vi "ep_Detect Signaling Voltage.vi"(7 "signaling frequency":dbl=216.66, 8 "error in (no error)":errorcluster, 10 "current spectrum (5Hz step)":T2, 11 "voltage spectrum (5Hz step)":T2) -> (0 "error out":errorcluster, 1 "detected signaling frequency [Hz]":dbl, 2 "signaling current RMS [A]":dbl, 3 "signaling voltage RMS [V]":dbl)   [LabVIEW 2014, in "NI_EP_Power Quality.lvlib"]
uses:
  <vilib>/addons/Electrical Power/PQ/NI_EP_Power Quality.lvlib
  <vilib>/addons/Electrical Power/PQ/Common/Controls/ep_AI Data Channel.ctl
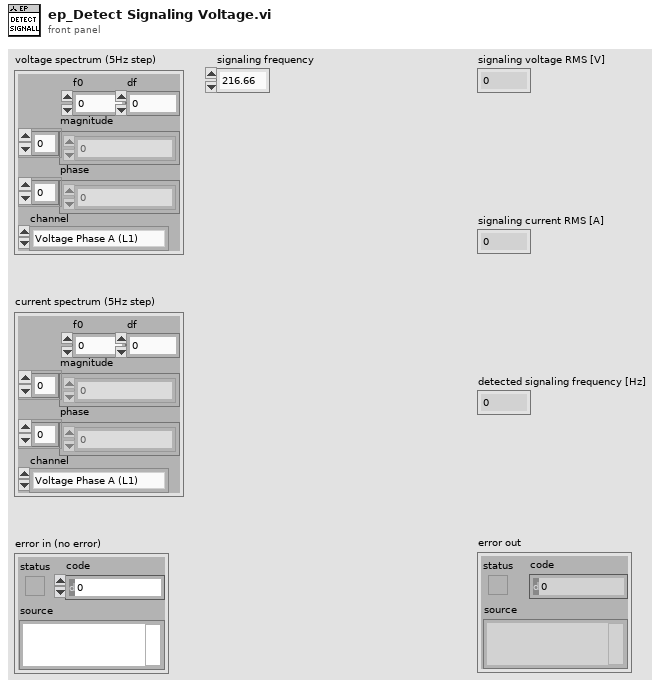
[diagram p1: front panel]
types:
  T1 = typedef "NI_EP_Power Quality.lvlib/ep_AI Data Channel.ctl" = enum16{"Voltage Phase A (L1)", "Voltage Phase B (L2)", "Voltage Phase C (L3)", "Voltage Phase N (Neutral)", "Current Phase A (L1)", "Current Phase B (L2)", "Current Phase C (L3)", "Current Phase N (Neutral)"}
  T2 = cluster{"f0":dbl, "df":dbl, "magnitude":dbl[], "phase":dbl[], "channel":T1}
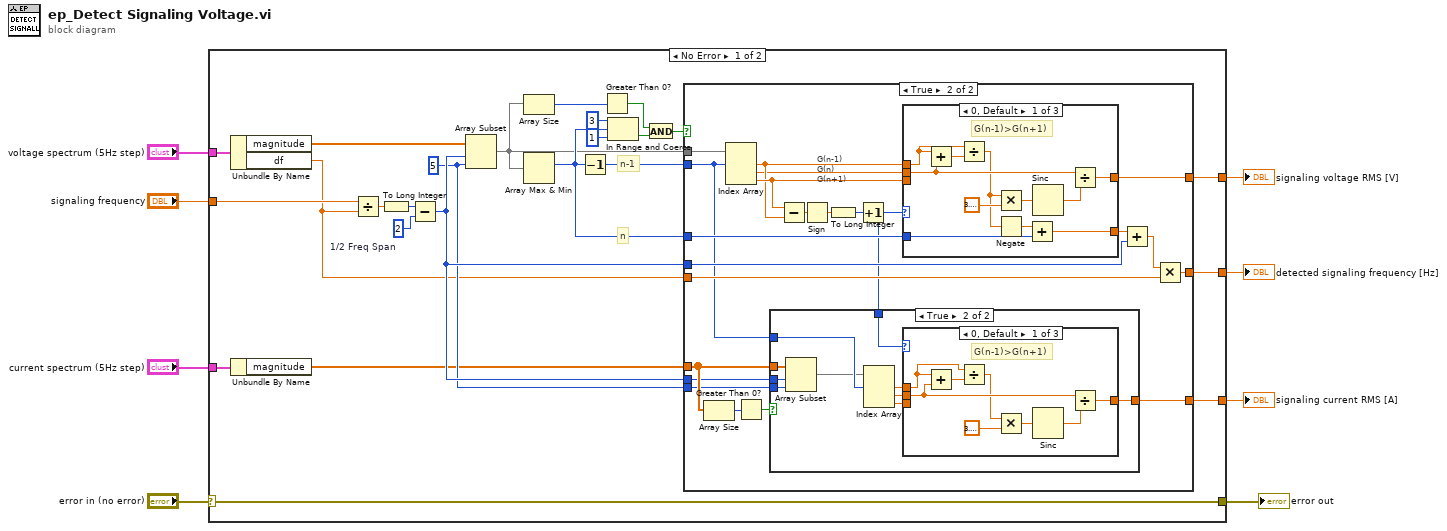
[diagram p0: block diagram]
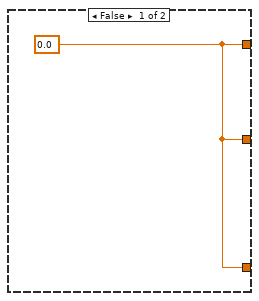
[diagram p2: hidden frame]
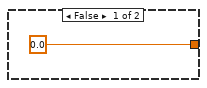
[diagram p3: hidden frame]
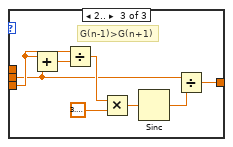
[diagram p5: hidden frame]
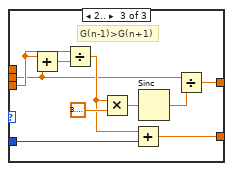
[diagram p7: hidden frame]
diagram:
  n1 = case shown="No Error" "error in (no error)" {
    selector: "error in (no error)" -> [w9 w107]
    tunnel: "current spectrum (5Hz step)" -> [w27 _]
    tunnel: "voltage spectrum (5Hz step)" -> [w26 _]
    tunnel: "signaling frequency" -> [w25 _]
    tunnel: [w24 _] -> w5
    tunnel: [w16 _] -> w4
    tunnel: [w14 _] -> w3
    tunnel: [w9 w107] -> w1
    frame No Error {
      w17 = 5 ("32bit integer")
      w31 = 2  # 1/2 Freq Span
      # "n"
      # "n-1"
      n2 = Unbundle By Name(w26) -> ("magnitude"=w12:dbl[], "df"=w15:dbl)
      n3 = Unbundle By Name(w27) -> ("magnitude"=w11:dbl[])
      n4 = Divide(x=w25, y=w15) -> (x/y=w13:dbl)
      n5 = To Long Integer(number=w13) -> (32bit integer=w32:i32)
      n6 = Subtract(x=w32, y=w31) -> (x-y=w18:i32)
      n7 = Array Subset(array=w12, index=w18, length=w17) -> (w10:dbl[])
      n8 = Array Size(array=w10) -> (size(s)=w29:i32)
      n9 = Array Max & Min(array=w10) -> (max index (indices)=w22:i32)  [unwired: 3 out]
      n10 = Decrement(x=w22) -> (x-1=w30:i32)
      n11 = Greater Than 0?(x=w29) -> (x > 0?=w23:bool)
      n12 = In Range and Coerce(upper limit=3, x=w22, lower limit=1) -> (In Range?=w19:bool)  [unwired: 1 out]
      n13 = And(x=w23, y=w19) -> (x .and. y?=w28:bool)
      n14 = case shown="True" w28 {
        tunnel: w30 -> [_ w35]
        tunnel: w15 -> [_ w55]
        tunnel: w10 -> [_ w45]
        tunnel: w18 -> [_ w46]
        tunnel: w22 -> [_ w54]
        tunnel: [w33 w51] -> w14
        tunnel: [w33 w48] -> w24
        tunnel: w11 -> [_ w38]
        tunnel: w18 -> [_ w37]
        tunnel: w17 -> [_ w36]
        tunnel: [w33 w34] -> w16
        frame False {
          w33 = 0.0
        }
        frame True {
          # "G(n-1)\nG(n)\nG(n+1)"
          n15 = Array Size(array=w38) -> (size(s)=w41:i32)
          n16 = Index Array(array=w45, index #1=w35) -> (element #1=w43:dbl, element #2=w42:dbl, element #3=w44:dbl)  [unwired: 2 in]
          n17 = Greater Than 0?(x=w41) -> (x > 0?=w40:bool)
          n18 = Subtract(x=w44, y=w43) -> (x-y=w52:dbl)
          n19 = Sign(1:w52) -> (0:w53:dbl)
          n20 = To Long Integer(number=w53) -> (32bit integer=w47:i32)
          n21 = Increment(x=w47) -> (x+1=w39:i32)
          n22 = case shown="True" w40 {
            tunnel: w39 -> [_ w59]
            tunnel: w38 -> [_ w66]
            tunnel: w37 -> [_ w65]
            tunnel: w36 -> [_ w64]
            tunnel: w35 -> [_ w63]
            tunnel: [0.0 ("vector") w58] -> w34
            frame False {
            }
            frame True {
              n23 = Array Subset(array=w66, index=w65, length=w64) -> (w57:dbl[])
              n24 = Index Array(array=w57, index #1=w63) -> (element #1=w62:dbl, element #2=w61:dbl, element #3=w60:dbl)  [unwired: 2 in]
              n25 = case shown="0, Default" w59 {
                tunnel: w60 -> [_ _ w79]
                tunnel: w62 -> [w72 _ _]
                tunnel: w61 -> [w70 w75 w76]
                tunnel: [w73 w75 w82] -> w58
                frame 0, Default {
                  # "G(n-1)>G(n+1)"
                  n26 = Add(x=w72, y=w70) -> (x+y=w68:dbl)
                  n27 = Divide(x=w72, y=w68) -> (x/y=w67:dbl)
                  n28 = Multiply(x=w67, y=3.141592653589793) -> (x*y=w71:dbl)
                  n29 = Sinc(1:w71) -> (0:w69:dbl)
                  n30 = Divide(x=w70, y=w69) -> (x/y=w73:dbl)
                }
                frame 1 {
                  # "G(n-1)=G(n+1)"
                }
                frame 2.. {
                  # "G(n-1)>G(n+1)"
                  n31 = Add(x=w79, y=w76) -> (x+y=w78:dbl)
                  n32 = Divide(x=w79, y=w78) -> (x/y=w77:dbl)
                  n33 = Multiply(x=w77, y=3.141592653589793) -> (x*y=w81:dbl)
                  n34 = Sinc(1:w81) -> (0:w80:dbl)
                  n35 = Divide(x=w76, y=w80) -> (x/y=w82:dbl)
                }
              }
            }
          }
          n36 = case shown="0, Default" w39 {
            tunnel: w44 -> [_ _ w100]
            tunnel: w43 -> [w90 _ _]
            tunnel: w42 -> [w87 w95 w97]
            tunnel: [w91 w96 w103] -> w50
            tunnel: [w93 w95 w105] -> w48
            tunnel: w54 -> [w92 w96 w104]
            frame 0, Default {
              # "G(n-1)>G(n+1)"
              n37 = Add(x=w90, y=w87) -> (x+y=w85:dbl)
              n38 = Divide(x=w90, y=w85) -> (x/y=w84:dbl)
              n39 = Multiply(x=w84, y=3.141592653589793) -> (x*y=w88:dbl)
              n40 = Negate(x=w84) -> (-x=w89:dbl)
              n41 = Add(x=w89, y=w92) -> (x+y=w91:dbl)
              n42 = Sinc(1:w88) -> (0:w86:dbl)
              n43 = Divide(x=w87, y=w86) -> (x/y=w93:dbl)
            }
            frame 1 {
              # "G(n-1)=G(n+1)"
            }
            frame 2.. {
              # "G(n-1)>G(n+1)"
              n44 = Add(x=w100, y=w97) -> (x+y=w99:dbl)
              n45 = Divide(x=w100, y=w99) -> (x/y=w98:dbl)
              n46 = Multiply(x=w98, y=3.141592653589793) -> (x*y=w102:dbl)
              n47 = Add(x=w98, y=w104) -> (x+y=w103:dbl)
              n48 = Sinc(1:w102) -> (0:w101:dbl)
              n49 = Divide(x=w97, y=w101) -> (x/y=w105:dbl)
            }
          }
          n50 = Add(x=w50, y=w46) -> (x+y=w49:dbl)
          n51 = Multiply(x=w49, y=w55) -> (x*y=w51:dbl)
        }
      }
    }
    frame Error {
    }
  }
  "signaling voltage RMS [V]" <- w5
  "signaling current RMS [A]" <- w4
  "detected signaling frequency [Hz]" <- w3
  "error out" <- w1
